vi "Display Image in Image Control.vi"(8 "Error In":errorcluster, 9 "Image to Display":T1, 11 "Display Image Control Refnum":T2) -> (0 "Error Out":errorcluster, 1 "Image Display Range":cluster{"Min Value":dbl, "Max Value":dbl}={"Min Value"=nan, "Max Value"=nan})   [LabVIEW 2021, in "Image.lvlib"]
uses:
  Image Control Refnum.ctl
  <vilib>/vision/Image Controls.llb/IMAQ Image.ctl
  Image.lvlib
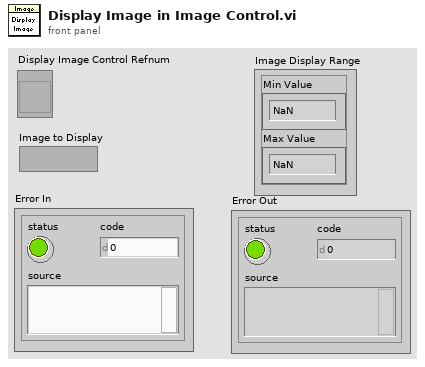
[diagram p1: front panel]
types:
  T1 = typedef "IMAQ Image.ctl" = refnum<image>
  T2 = typedef "Image.lvlib/Image Control Refnum.ctl" = refnum<vi>
  T3 = typedef "Image Type" = u32
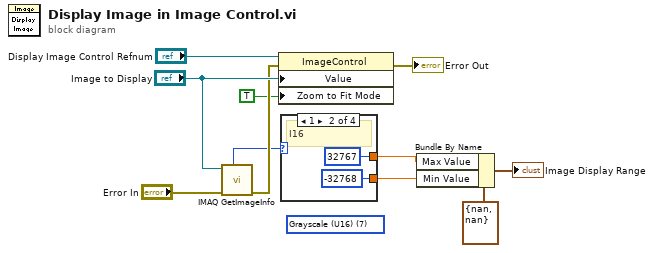
[diagram p0: block diagram]
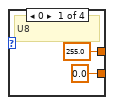
[diagram p2: hidden frame]
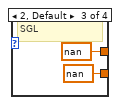
[diagram p3: hidden frame]
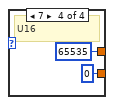
[diagram p4: hidden frame]
diagram:
  (unwired) T3 7 items=["Grayscale (U8)", "Grayscale (I16)", "Grayscale (SGL)", "Complex (CSG)", "RGB (U32)", "HSL (U32)", "RGB (U64)", "Grayscale (U16)"] ("Image Type")
  n1 = call "IMAQ GetImageInfo"("error in (no error)"="Error In", "Image"="Image to Display") -> ("error out"=w7:errorcluster, "Image Type"=w6:T3)  [unwired: 2 in, 6 out]
  n2 = property class="ImageControl"(reference="Display Image Control Refnum", error in=w7, "Value"="Image to Display", "Zoom to Fit Mode"=TRUE) -> (error out=→"Error Out":errorcluster)  [unwired: 1 out]
  n3 = case shown="1" w6 {
    tunnel: [255.0 ("Display max") i16 32767 ("Display max") sgl nan ("Display max") u16 65535 ("Display max")] -> w5
    tunnel: [0.0 ("Display min") i16 -32768 ("Display max") sgl nan ("Display max") u16 0 ("Display max")] -> w4
    frame 0 {
      # "U8"
    }
    frame 1 {
      # "I16"
    }
    frame 2, Default {
      # "SGL"
    }
    frame 7 {
      # "U16"
    }
  }
  n4 = Bundle By Name(cluster=cluster{"Min Value":dbl, "Max Value":dbl} {"Min Value"=nan, "Max Value"=nan} ("Image Display Range"), "Max Value"=w5, "Min Value"=w4) -> (→"Image Display Range":cluster{"Min Value":dbl, "Max Value":dbl})
